vi "SET_DAC.vi"(8 "error in (no error)":errorcluster, 10 "DAC value":ext caption="DAC Value", 11 "VISA Refnum in":refnum<visa-resource-name>) -> (0 "error out":errorcluster, 3 "VISA Refnum out":refnum<visa-resource-name>)   [LabVIEW 2019]
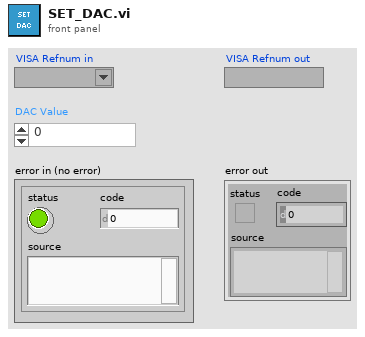
[diagram p1: front panel]
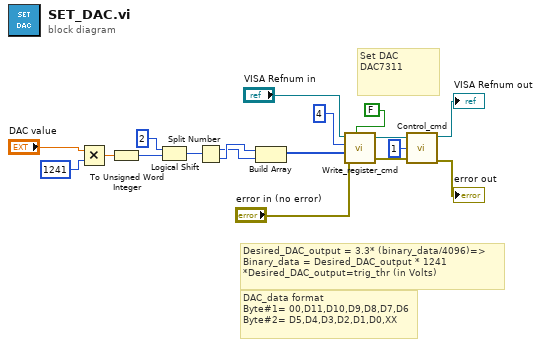
[diagram p0: block diagram]
diagram:
  # "DAC_data format\nByte#1= 00,D11,D10,D9,D8,D7,D6\nByte#2= D5,D4,D3,D2,D1,D0,XX"
  # "Desired_DAC_output = 3.3* (binary_data/4096)=>\nBinary_data = Desired_DAC_output * 1241\n*Desired_DAC_output=trig_thr (in Volts)"
  # "Set DAC\nDAC7311"
  n1 = Multiply(x="DAC value", y=1241) -> (x*y=w3:ext)
  n2 = To Unsigned Word Integer(number=w3) -> (unsigned 16bit integer=w4:u16)
  n3 = Logical Shift(y=i16 2, x=w4) -> (x << y=w5:u16)
  n4 = Split Number(x=w5) -> (hi(x)=w12:u8, lo(x)=w13:u8)
  n5 = Build Array(w13, w12) -> (w10:u8[])
  n6 = call "Write_register_cmd.vi"("Fifo-mode En"=FALSE, "Arty-7 Error In"="error in (no error)", "Data Array"=w10, "WrReg Addr"=u8 4 ("WrReg Address 2"), "Arty-7 VISA In"="VISA Refnum in") -> ("Arty-7 Error out"=w8:errorcluster, "Arty-7 VISA out"=w9:refnum<visa-resource-name>)  [unwired: 3 in, 2 out]
  n7 = call "Control_cmd.vi"("Arty-7 Error In"=w8, "Control Command"=u8 1, "Arty-7 VISA In"=w9) -> ("Arty-7 Error out"=→"error out":errorcluster, "Arty-7 VISA out"=→"VISA Refnum out":refnum<visa-resource-name>)  [unwired: 2 in, 2 out]
